vi "open_plot_and_find_double_peak.vi"() -> ()   [LabVIEW 2013]
uses:
  Classes/Plots/Plots.lvclass
  <vilib>/Utility/file.llb/Read From Spreadsheet File (string).vi
  global variables.vi
  MSEval/global_variables.vi
panel:
  in  "file path (dialog if empty)":path=path "C:/Users/Thermo/Documents/GitHub/HelixMC/MSControl/test_vis/double_peak_data_full.txt"
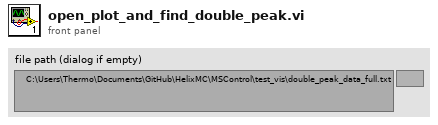
[diagram p1: front panel]
types:
  T1 = cluster{"format string":string, "Variant":variant}
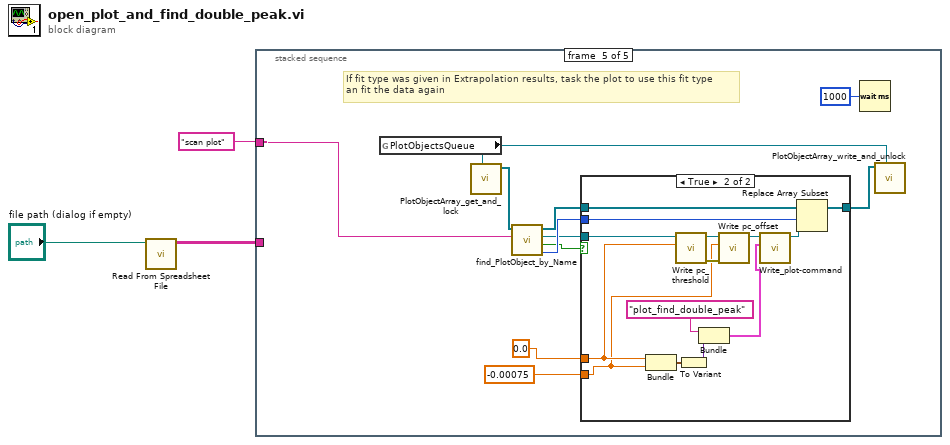
[diagram p0: block diagram]
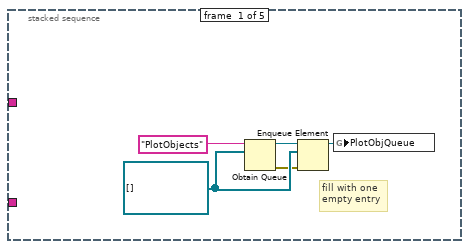
[diagram p2: hidden frame]
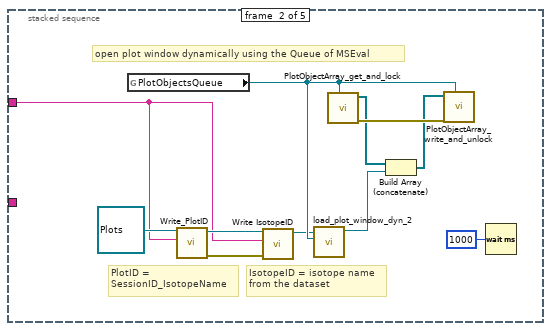
[diagram p3: hidden frame]
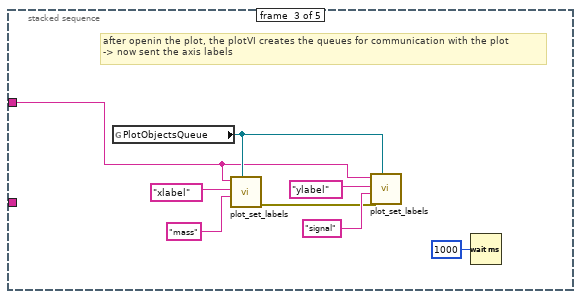
[diagram p4: hidden frame]
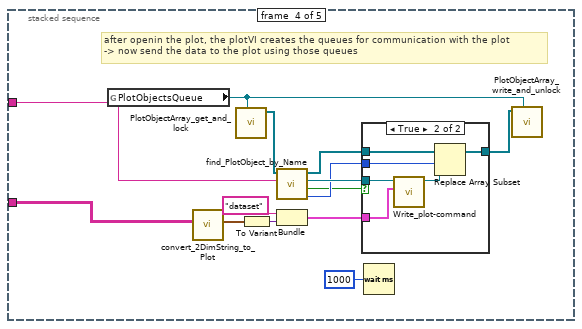
[diagram p5: hidden frame]
diagram:
  n1 = call-poly <vilib>:"Read From Spreadsheet File.vi"("file path (dialog if empty)"="file path (dialog if empty)") -> ("all rows"=w1:string[][])  [unwired: 6 in, 4 out]
  n2 = stacked-sequence {
    tunnel: "scan plot" -> [_ w10 w21 w31 w52]
    tunnel: w1 -> [_ _ _ w29 _]
    frame #0 {
      w6 = refnum<class "Plots.lvclass">[] [] ("PlotObjArray")
      # "fill with one\nempty entry"
      n3 = Obtain Queue(name (unnamed)="PlotObjects", element data type=w6) -> (queue out=w7:refnum<queue>, error out=w4:errorcluster)  [unwired: 3 in, 1 out]
      n4 = Enqueue Element(queue=w7, element=w6, error in (no error)=w4) -> (queue out=w5:refnum<queue>)  [unwired: 1 in, 2 out]
      n5 = global write "global variables.vi" "PlotObjQueue"(w5) -> ()
    }
    frame #1 {
      # "IsotopeID = isotope name\nfrom the dataset"
      # "PlotID =\nSessionID_IsotopeName"
      # "open plot window dynamically using the Queue of MSEval"
      n6 = global read "global_variables.vi" "PlotObjectsQueue"() -> (w14:refnum<queue>)
      n7 = call-dynamic "Write_PlotID.vi"("PlotID"=w10, "Plots in"=refnum<class "Plots.lvclass"> refnum ("Plots.lvclass")) -> ("error out"=w12:errorcluster, "Plots out"=w13:refnum<class "Plots.lvclass">)  [unwired: 8 in]
      n8 = call-dynamic "Write IsotopeID.vi"("error in (no error)"=w12, "IsotopeID"=w10, "Plots in"=w13) -> ("Plots out"=w11:refnum<class "Plots.lvclass">)  [unwired: 7 in, 1 out]
      n9 = call "load_plot_window_dyn_2.vi"("Ext PlotObjQueue in"=w14, "Plots in"=w11) -> ("Plots out"=w16:refnum<class "Plots.lvclass">)  [unwired: 8 in, 1 out]
      n10 = call "PlotObjectArray_get_and_lock.vi"("External PlotObjQueue in"=w14) -> ("error out"=w19:errorcluster, "PlotObjects"=w17:refnum<class "Plots.lvclass">[])  [unwired: 9 in]
      n11 = Build Array (concatenate)(w17, w16) -> (w15:refnum<class "Plots.lvclass">[])
      n12 = call "PlotObjectArray_write_and_unlock.vi"("External PlotObjQueue in"=w14, "error in (no error)"=w19, "PlotObjects"=w15) -> ()  [unwired: 8 in, 1 out]
      n13 = Wait (ms)(milliseconds to wait=u32 1000) -> ()  [unwired: 1 out]
    }
    frame #2 {
      # "after openin the plot, the plotVI creates the queues for communication with the plot\n-> now sent the axis labels"
      n14 = global read "global_variables.vi" "PlotObjectsQueue"() -> (w22:refnum<queue>)
      n15 = call "plot_set_labels.vi"("External PlotObjQueue in"=w22, "label"="mass", "axis"="xlabel", "plot name"=w21) -> ("error out"=w23:errorcluster)  [unwired: 7 in]
      n16 = call "plot_set_labels.vi"("External PlotObjQueue in"=w22, "error in (no error)"=w23, "label"="signal", "axis"="ylabel", "plot name"=w21) -> ()  [unwired: 6 in, 1 out]
      n17 = Wait (ms)(milliseconds to wait=u32 1000) -> ()  [unwired: 1 out]
    }
    frame #3 {
      # "after openin the plot, the plotVI creates the queues for communication with the plot\n-> now send the data to the plot using those queues"
      n18 = global read "global_variables.vi" "PlotObjectsQueue"() -> (w41:refnum<queue>)
      n19 = call "convert_2DimString_to_Plot.vi"("string data in"=w29) -> ("Plot Data"=w33:cluster{dbl, dbl, "flag":u8}[])  [unwired: 9 in, 1 out]
      n20 = call "PlotObjectArray_get_and_lock.vi"("External PlotObjQueue in"=w41) -> ("PlotObjects"=w40:refnum<class "Plots.lvclass">[])  [unwired: 9 in, 1 out]
      n21 = To Variant(anything=w33) -> (Variant=w34:variant)
      n22 = call "find_PlotObject_by_Name.vi"("Plot Name/ID"=w31, "PlotObj Array in"=w40) -> ("index of Object in Array"=w38:i32, "found?"=w30:bool, "found PlotObj out"=w39:refnum<class "Plots.lvclass">, "PlotObj Array out"=w37:refnum<class "Plots.lvclass">[])  [unwired: 6 in]
      n23 = Bundle("format string"="dataset", "Variant"=w34) -> (w32:T1)  [unwired: 1 in]
      n24 = case shown="True" w30 {
        tunnel: w39 -> [_ w48]
        tunnel: w38 -> [_ w46]
        tunnel: w37 -> [w42 w45]
        tunnel: [w42 w44] -> w36
        tunnel: w32 -> [_ w43]
        frame False {
        }
        frame True {
          n25 = call-dynamic "Write_plot-command.vi"("plot command"=w43, "Plots in"=w48) -> ("Plots out"=w47:refnum<class "Plots.lvclass">)  [unwired: 8 in, 1 out]
          n26 = Replace Array Subset(array=w45, new element=w47, index=w46) -> (w44:refnum<class "Plots.lvclass">[])
        }
      }
      n27 = Wait (ms)(milliseconds to wait=u32 1000) -> ()  [unwired: 1 out]
      n28 = call "PlotObjectArray_write_and_unlock.vi"("External PlotObjQueue in"=w41, "PlotObjects"=w36) -> ()  [unwired: 9 in, 1 out]
    }
    frame #4 {
      # "If fit type was given in Extrapolation results, task the plot to use this fit type\nan fit the data again"
      n29 = global read "global_variables.vi" "PlotObjectsQueue"() -> (w59:refnum<queue>)
      n30 = call "PlotObjectArray_get_and_lock.vi"("External PlotObjQueue in"=w59) -> ("PlotObjects"=w58:refnum<class "Plots.lvclass">[])  [unwired: 9 in, 1 out]
      n31 = call "find_PlotObject_by_Name.vi"("Plot Name/ID"=w52, "PlotObj Array in"=w58) -> ("index of Object in Array"=w57:i32, "found?"=w53:bool, "found PlotObj out"=w54:refnum<class "Plots.lvclass">, "PlotObj Array out"=w56:refnum<class "Plots.lvclass">[])  [unwired: 6 in]
      n32 = case shown="True" w53 {
        tunnel: w57 -> [_ w73]
        tunnel: w56 -> [w60 w72]
        tunnel: [w60 w71] -> w55
        tunnel: w54 -> [_ w68]
        tunnel: 0.0 -> [_ w62]
        tunnel: -0.00075 -> [_ w61]
        frame False {
        }
        frame True {
          n33 = Bundle(w62, w61) -> (w66:cluster{dbl, dbl})  [unwired: 1 in]
          n34 = call-dynamic "Write pc_threshold.vi"("pc_threshold"=w62, "Plots in"=w68) -> ("error out"=w69:errorcluster, "Plots out"=w70:refnum<class "Plots.lvclass">)  [unwired: 8 in]
          n35 = To Variant(anything=w66) -> (Variant=w65:variant)
          n36 = Bundle("format string"="plot_find_double_peak", "Variant"=w65) -> (w63:T1)  [unwired: 1 in]
          n37 = call-dynamic "Write pc_offset.vi"("error in (no error)"=w69, "pc_offset"=w61, "Plots in"=w70) -> ("Plots out"=w67:refnum<class "Plots.lvclass">)  [unwired: 7 in, 1 out]
          n38 = call-dynamic "Write_plot-command.vi"("plot command"=w63, "Plots in"=w67) -> ("Plots out"=w74:refnum<class "Plots.lvclass">)  [unwired: 8 in, 1 out]
          n39 = Replace Array Subset(array=w72, new element=w74, index=w73) -> (w71:refnum<class "Plots.lvclass">[])
        }
      }
      n40 = Wait (ms)(milliseconds to wait=u32 1000) -> ()  [unwired: 1 out]
      n41 = call "PlotObjectArray_write_and_unlock.vi"("External PlotObjQueue in"=w59, "PlotObjects"=w55) -> ()  [unwired: 9 in, 1 out]
    }
  }
